vi "模式匹配.vi"() -> ()   [LabVIEW 2012]
uses:
  halcondotnet.dll
panel:
  out "find":dbl[](array[numeric])
  in  "路径":path
  in  "HWindowControl":refnum<k24>(container)
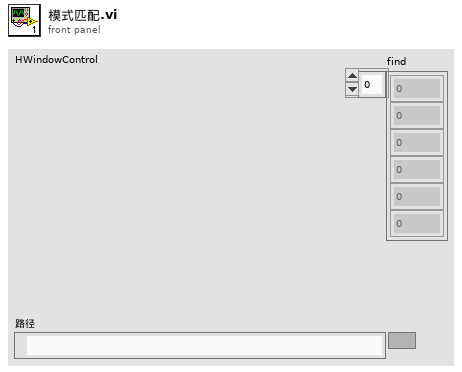
[diagram p1: front panel]
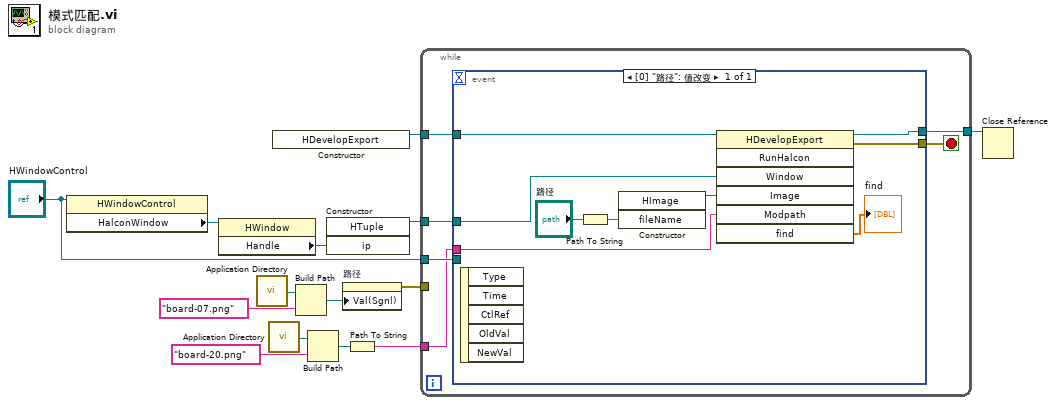
[diagram p0: block diagram]
diagram:
  n1 = property class="HWindowControl"(reference="HWindowControl") -> ("HalconWindow"=w7:refnum<k24>)  [unwired: 1 in, 2 out]
  n2 = property class="HWindow"(reference=w7) -> ("Handle"=w6:refnum<k24>)  [unwired: 1 in, 2 out]
  n3 = call <vilib>:"Application Directory.vi"() -> ("Application Directory"=w13:path)
  n4 = call <vilib>:"Application Directory.vi"() -> ("Application Directory"=w3:path)
  n5 = constructor class="HDevelopExport"() -> (reference out=w14:refnum<k24>)  [unwired: 3 in, 2 out]
  n6 = Build Path(base path=w13, name or relative path="board-07.png" ("名称或相对路径")) -> (appended path=w10:path)
  n7 = Build Path(base path=w3, name or relative path="board-20.png" ("名称或相对路径")) -> (appended path=w2:path)
  n8 = constructor class="HTuple"("ip"=w6) -> (reference out=w5:refnum<k24>)  [unwired: 3 in, 3 out]
  n9 = property on="路径" class="Path"("Val(Sgnl)"=w10) -> (error out=w11:errorcluster)  [unwired: 2 in, 1 out]
  n10 = Path To String(path=w2) -> (string=w1:string)
  n11 = while {
    tunnel: w14 -> [w20]
    tunnel: "HWindowControl" -> [w19]
    tunnel: w11 -> [_]
    tunnel: [w17] -> w9
    tunnel: w5 -> [w16]
    tunnel: w1 -> [w15]
    stop <- w18 stop-if-true
    n12 = event shown="[0] \"路径\": 值改变" {
      selector: _ -> [_]
      dyn-events: _ -> [_]
      timeout: _ -> [_]
      tunnel: w20 -> [w29]
      tunnel: w19 -> [_]
      tunnel: [w25] -> w18
      tunnel: [w24] -> w17
      tunnel: w16 -> [w23]
      tunnel: w15 -> [w21]
      event "路径": Value Change {
        n13 = event-data() -> ()  [unwired: 1 in, 5 out]
        n14 = Path To String(path="路径") -> (string=w27:string)
        n15 = constructor class="HImage"("fileName"=w27) -> (reference out=w28:refnum<k24>)  [unwired: 3 in, 3 out]
        n16 = invoke class="HDevelopExport" method="RunHalcon"(reference=w29, "Window"=w23, "Image"=w28, "Modpath"=w21) -> (reference out=w24:refnum<k24>, error out=w25:errorcluster, "find"=→"find":dbl[])  [unwired: 3 in, 4 out]
      }
    }
  }
  n17 = Close Reference(reference=w9) -> ()  [unwired: 1 in, 1 out]
